vi "Configure Arbitrary Waveform Frequency.vi"(8 "error in (no error)":errorcluster, 9 "Arbitrary Waveform Frequency (1000 Hz)":dbl=1000.0 format="%#.4f", 10 "Channel (1: 1)":i32(ring)=1 items=["1"=1, "2"=2], 11 "VISA resource name":refnum<visa-resource-name>) -> (0 "error out":errorcluster, 3 "VISA resource name out":refnum<visa-resource-name>)   [LabVIEW 2019, in "Agilent 3352X Series.lvlib"]
doc: "Configures for the frequency of the arbitrary waveform."
uses:
  Agilent 3352X Series.lvlib
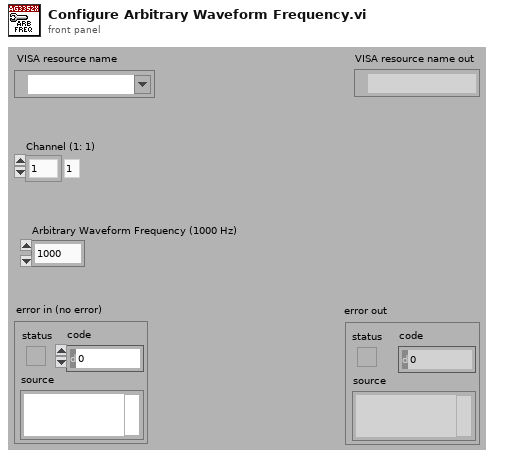
[diagram p1: front panel]
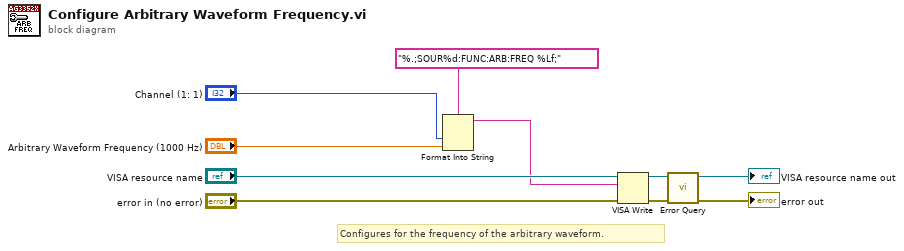
[diagram p0: block diagram]
diagram:
  # "Configures for the frequency of the arbitrary waveform."
  n1 = Format Into String(format string="%.;SOUR%d:FUNC:ARB:FREQ %Lf;", "Channel (1: 1)", "Arbitrary Waveform Frequency (1000 Hz)") -> (resulting string=w1:string)  [unwired: 2 in, 1 out]
  n2 = VISA Write(VISA resource name="VISA resource name", write buffer=w1, error in (no error)="error in (no error)") -> (VISA resource name out=w6:refnum<visa-resource-name>, error out=w5:errorcluster)  [unwired: 1 out]
  n3 = call "Error Query.vi"("error in (no error)"=w5, "VISA resource name"=w6) -> ("error out"=→"error out":errorcluster, "VISA resource name out"=→"VISA resource name out":refnum<visa-resource-name>)  [unwired: 8 out]
